vi "Configure System Time.vi"(7 "Second (0)":i32, 8 "error in (no error)":errorcluster, 9 "Minute (0)":i32, 10 "Hour (0)":i32, 11 "VISA resource name":refnum<visa-resource-name>) -> (0 "error out":errorcluster, 3 "VISA resource name out":refnum<visa-resource-name>)   [LabVIEW 2020, in "Rohde&Schwarz CMXP Base.lvlib"]
doc: "Sets the universal time coordinated (UTC) of the operating system clock.\n\nAttribute:\n-\n\nRemote-control command:\nSYSTem:TIME[:UTC]"
uses:
  <instrlib>/Rohde&Schwarz CMXP Base/Rohde&Schwarz CMXP Base.lvlib
  <instrlib>/Rohde&Schwarz CMXP Base/Private/rsidr_core.llb/rsidr_core.lvlib
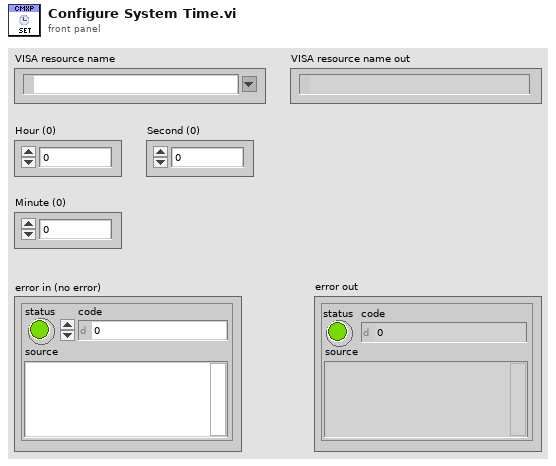
[diagram p1: front panel]
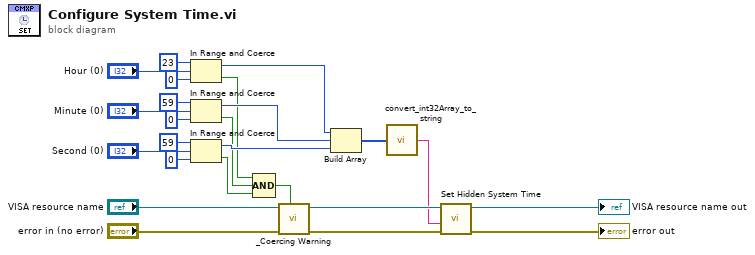
[diagram p0: block diagram]
diagram:
  n1 = In Range and Coerce(upper limit=23, x="Hour (0)", lower limit=0) -> (coerced(x)=w8:i32, In Range?=w2:bool)
  n2 = In Range and Coerce(upper limit=59, x="Minute (0)", lower limit=0) -> (coerced(x)=w7:i32, In Range?=w3:bool)
  n3 = In Range and Coerce(upper limit=59, x="Second (0)", lower limit=0) -> (coerced(x)=w6:i32, In Range?=w4:bool)
  n4 = Compound Arithmetic op=AND(w2, w3, w4) -> (w11:bool)
  n5 = call <instrlib>:"_Coercing Warning.vi"("In Range?"=w11, "error in (no error)"="error in (no error)", "VISA resource name"="VISA resource name") -> ("error out"=w9:errorcluster, "VISA resource name out"=w10:refnum<visa-resource-name>)  [unwired: 7 in]
  n6 = Build Array(w8, w7, w6) -> (w5:i32[])
  n7 = call <instrlib>:"convert_int32Array_to_string.vi"("I32 array in"=w5) -> ("string out"=w1:string)  [unwired: 4 in]
  n8 = call "Set Hidden System Time"("error in (no error)"=w9, "Hidden System Time ()"=w1, "instrument handle"=w10) -> ("error out"=→"error out":errorcluster, "instrument handle out"=→"VISA resource name out":refnum<visa-resource-name>)  [unwired: 7 in]
